vi "TDC_setHbtInput.vi"(8 "Error In":errorcluster, 10 "Channel 2":i32=100, 11 "Channel 1":i32=2) -> (0 "Error Out":errorcluster)   [LabVIEW 2011]
uses:
  tdcbase.dll
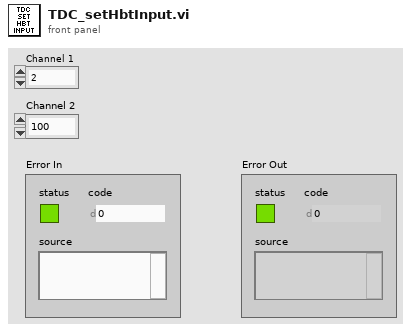
[diagram p1: front panel]
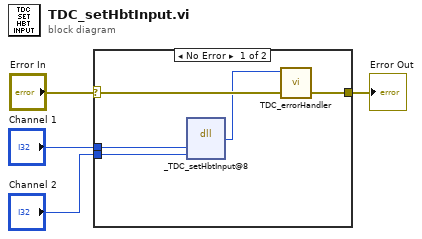
[diagram p0: block diagram]
diagram:
  n1 = case shown="No Error" "Error In" {
    selector: "Error In" -> [w8 w10]
    tunnel: [w7 w10] -> w3
    tunnel: "Channel 1" -> [w9 _]
    tunnel: "Channel 2" -> [w6 _]
    frame No Error {
      n2 = dll-call lib="X:/tdcbase.dll" fn="_TDC_setHbtInput@8"("channel1"=w9, "channel2"=w6) -> ("return type"=w5:i32)  [unwired: 5 in, 2 out]
      n3 = call "TDC_errorHandler.vi"("Error In"=w8, "TDC Return Code"=w5) -> ("Error Out"=w7:errorcluster)  [unwired: 9 in]
    }
    frame Error {
    }
  }
  "Error Out" <- w3
